vi "Excersie_7.vi"() -> ()   [LabVIEW 2013]
doc: "Use this template to build a standard state machine design pattern. Each state executes code and determines which state to transition to. Contrast this design pattern with the User Interface Event Handler pattern, in which code executes in response to user actions. Contrast this design pattern also with the Queued Message Handler pattern, in which each message handling code can queue zero or more new messages.\nNote: This template does not contain the most recent programming guidelines recommended by National Instruments. For a complete, project-based implementation of the Standard State Machine pattern, use the Create Project dialog box instead of this template."
uses:
  StateMachineStates 1.ctl
panel:
  out "State":T1
  in  "Begin Test":bool
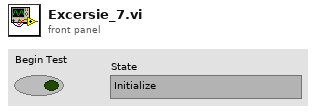
[diagram p1: front panel]
types:
  T1 = typedef "StateMachineStates 1.ctl" = enum16{"Initialize", "Idle", "Test", "Stop"}
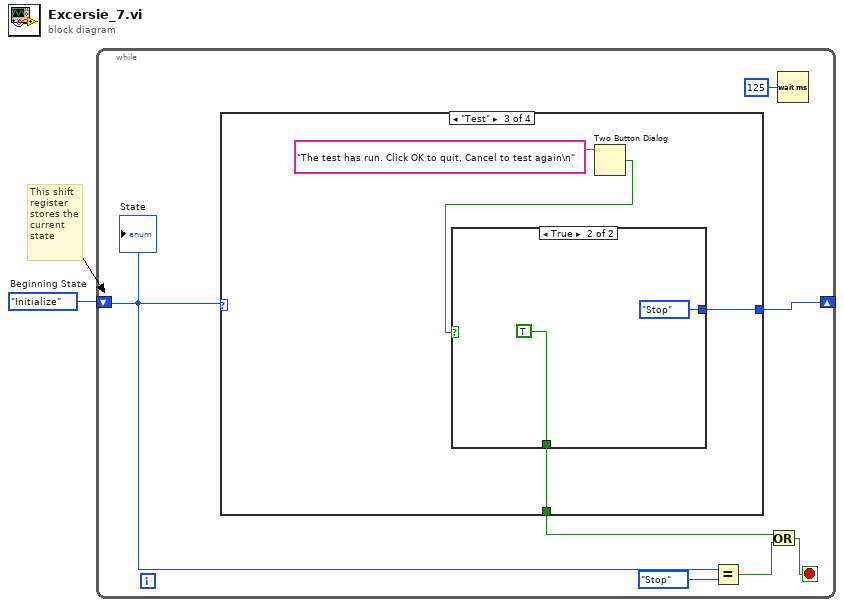
[diagram p0: block diagram]
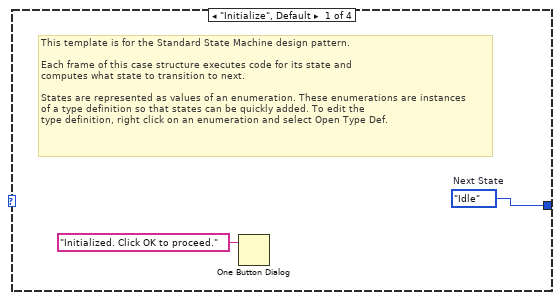
[diagram p2: hidden frame]
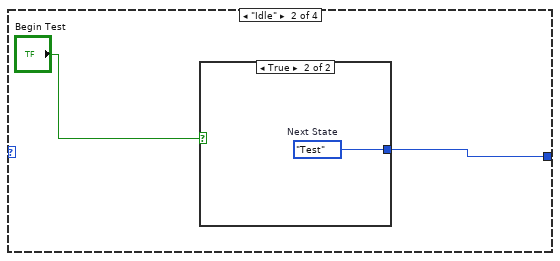
[diagram p3: hidden frame]
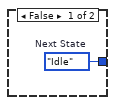
[diagram p4: hidden frame]
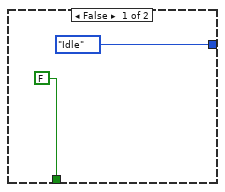
[diagram p5: hidden frame]
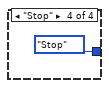
[diagram p6: hidden frame]
diagram:
  w1 = StateMachineStates_1."Initialize"  # Beginning State
  # "This shift\nregister\nstores the\ncurrent\nstate"
  n1 = while {
    shift-right: [w7] -> _
    shift-left: w1 -> [w2]
    stop <- w3 stop-if-true
    n2 = case shown="\"Test\"" w2 {
      tunnel: [w10 w12 w16 StateMachineStates_1."Stop" ("Next State")] -> w7
      tunnel: [_ _ w15 _] -> w5
      frame "Initialize", Default {
        w10 = StateMachineStates_1."Idle"  # Next State
        # "This template is for the Standard State Machine design pattern.\n\nEach frame of this case structure executes code for its state and\ncomputes what state to transition to next.\n\nStates are represented as values of an enumeration. These enumerations are instances\nof a type definition so that states can be quickly added. To edit the \ntype definition, right click on an enumeration and select Open Type Def."
        n3 = One Button Dialog(message="Initialized. Click OK to proceed.") -> ()  [unwired: 1 in, 1 out]
      }
      frame "Idle" {
        n4 = case shown="True" "Begin Test" {
          tunnel: [w13 w14] -> w12
          frame False {
            w13 = StateMachineStates_1."Idle"  # Next State
          }
          frame True {
            w14 = StateMachineStates_1."Test"  # Next State
          }
        }
      }
      frame "Test" {
        n5 = Two Button Dialog(message="The test has run. Click OK to quit, Cancel to test again\n") -> (T button?=w17:bool)  [unwired: 2 in]
        n6 = case shown="True" w17 {
          tunnel: [StateMachineStates_1."Idle" ("Next State") StateMachineStates_1."Stop" ("Next State")] -> w16
          tunnel: [FALSE TRUE] -> w15
          frame False {
          }
          frame True {
          }
        }
      }
      frame "Stop" {
      }
    }
    n7 = Equal?(x=w2, y=StateMachineStates_1."Stop" ("States")) -> (x = y?=w4:bool)
    n8 = Or(x=w5, y=w4) -> (x .or. y?=w3:bool)
    n9 = Wait (ms)(milliseconds to wait=u32 125) -> ()  [unwired: 1 out]
    "State" <- w2
  }
